vi "Prepare Control.vi"(7 "VolatusAPI":refnum<class "VolatusAPI.lvclass">, 8 "error in (no error)":errorcluster, 11 "ValveControl in":refnum<class "TimedPWMControl.lvclass">) -> (0 "error out":errorcluster, 3 "ValveControl out":refnum<class "TimedPWMControl.lvclass">)   [LabVIEW 2020, in "VolatusControl.lvlib" / "TimedPWMControl.lvclass"]
uses:
  TimedPWMControl.lvclass
  Volatus/VolatusAPI/VolatusAPI.lvclass
  TimedPWMControl.lvclass/TimedPWMControl.ctl
  lv-vecto/Vecto/Group/Group.lvclass
  lv-vecto/Vecto/GroupAbstract/GroupAbstract.lvclass
  C:/dev/lv20CE/relink/lv-vecto/Vecto/GroupAbstract/GroupAbstract.lvclass
  C:/dev/lv20CE/relink/lv-vecto/Vecto/Group/Group.lvclass
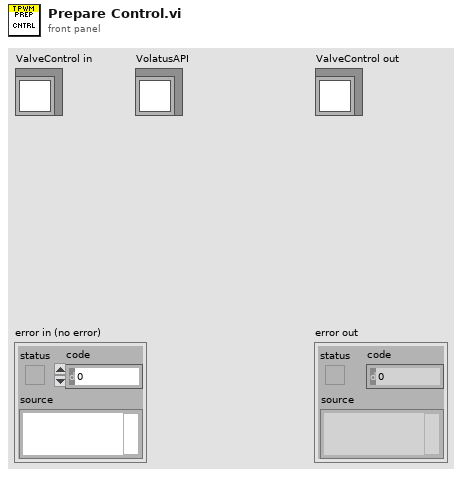
[diagram p1: front panel]
types:
  T1 = typedef "VectoConfig.lvlib/Channel Info.ctl" = cluster{"Name":string, "Group":string, "Owning Node":string, "Owning Task":string, "Resource":string}
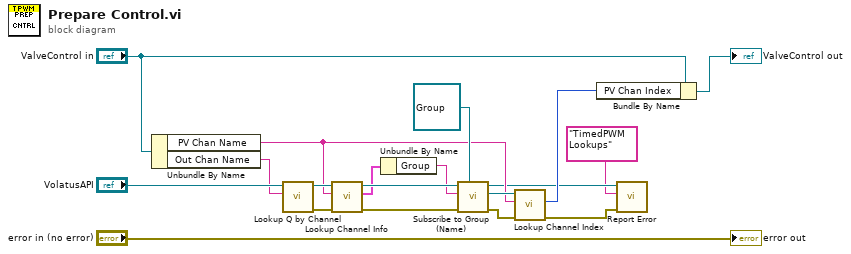
[diagram p0: block diagram]
diagram:
  n1 = Unbundle By Name("ValveControl in") -> ("PV Chan Name"=w6:string, "Out Chan Name"=w16:string)
  n2 = call "Lookup Q by Channel.vi"("Channel Name"=w16, "VolatusAPI in"="VolatusAPI") -> ("error out"=w11:errorcluster, "VolatusAPI out"=w15:refnum<class "VolatusAPI.lvclass">)  [unwired: 7 in, 1 out]
  n3 = call "Lookup Channel Info.vi"("error in (no error)"=w11, "Channel Name"=w6, "VolatusAPI in"=w15) -> ("error out"=w10:errorcluster, "Channel Info"=w9:T1, "VolatusAPI out"=w14:refnum<class "VolatusAPI.lvclass">)  [unwired: 5 in, 1 out]
  n4 = Unbundle By Name(w9) -> ("Group"=w13:string)
  n5 = call "Subscribe to Group (Name).vi"("Group Type"=refnum<class "Group.lvclass"> refnum ("Vecto.lvlib:Group.lvclass"), "error in (no error)"=w10, "Group Name"=w13, "VolatusAPI in"=w14) -> ("error out"=w7:errorcluster, "Group"=w8:refnum<class "Group.lvclass">, "VolatusAPI out"=w3:refnum<class "VolatusAPI.lvclass">)  [unwired: 5 in]
  n6 = call "Lookup Channel Index.vi"("error in (no error)"=w7, "Channel Name"=w6, "GroupAbstract in"=w8) -> ("error out"=w2:errorcluster, "Index"=w4:i32)  [unwired: 6 in, 1 out]
  n7 = Bundle By Name(cluster="ValveControl in", "PV Chan Index"=w4) -> (→"ValveControl out":refnum<class "TimedPWMControl.lvclass">)
  n8 = call "Report Error.vi"("error in (no error)"=w2, "Context"="TimedPWM Lookups", "VolatusAPI in"=w3) -> ()  [unwired: 7 in, 2 out]
  "error out" <- "error in (no error)"
